vi "DO COUNTER.vi"() -> ()   [LabVIEW 2015]
uses:
  <vilib>/myRIO/Instrument Drivers/Onboard IO/DIO/typedefs/DIO Reference.ctl
  <vilib>/myRIO/Common/Instrument Driver Framework/Utilities/typedefs/myRIO Generic Hardware Reference.ctl
  <vilib>/myRIO/Common/Instrument Driver Framework/Utilities/typedefs/Hardware Version Enum.ctl
  <vilib>/myRIO/Common/Instrument Driver Framework/Utilities/typedefs/myRIO v1.0 Reference.ctl
  <vilib>/myRIO/Common/Instrument Driver Framework/Utilities/typedefs/Generic FPGA Reference.ctl
  <vilib>/myRIO/Common/Instrument Driver Framework/myRIO v1.0/DIO/typedefs/DIO Channels List.ctl
  <vilib>/myRIO/Common/Instrument Driver Framework/myRIO v1.0/DIO/typedefs/DIO Channels Enum.ctl
  <vilib>/userdefined/High Color/nirio_resource_hc.ctl
  <vilib>/myRIO/Common/Instrument Driver Framework/Utilities/vis/Is FPGA Ref Available.vi
  <vilib>/myRIO/Common/Instrument Driver Framework/myRIO v1.0/DIO/vis/myRIO v1.1 Open DIO.vi
  <vilib>/myRIO/Instrument Drivers/Onboard IO/DIO/vis/Write.vi
  <vilib>/myRIO/Common/Instrument Driver Framework/Utilities/vis/Validate Channels.vi
  <vilib>/myRIO/Common/Instrument Driver Framework/myRIO v1.0/DIO/vis/myRIO v1.0 Reserve DIO.vi
  <vilib>/myRIO/Common/Instrument Driver Framework/myRIO v1.0/Resource Manager/vis/myRIO v1.0 Reserve Channel List.vi
  <vilib>/myRIO/Common/Instrument Driver Framework/myRIO v1.0/DIO/vis/myRIO v1.0 Build MUX Configuration DIO.vi
  <vilib>/myRIO/Common/Instrument Driver Framework/myRIO v1.0/Resource Manager/vis/myRIO v1.0 Reserve Channel.vi
  <vilib>/myRIO/Common/Instrument Driver Framework/myRIO v1.0/Resource Manager/vis/myRIO v1.0 Unreserve Channel.vi
  <vilib>/myRIO/Common/Instrument Driver Framework/myRIO v1.0/Resource Manager/vis/myRIO v1.0 Create Configuration List.vi
  <vilib>/myRIO/Common/Instrument Driver Framework/myRIO v1.0/Resource Manager/vis/myRIO v1.0 Build Mutex Name.vi
  <vilib>/Utility/VariantDataType/GetNumericInfo.vi
  <vilib>/Utility/error.llb/Error Cluster From Error Code.vi
  <vilib>/myRIO/Common/Instrument Driver Framework/myRIO v1.0/myRIO v1.1 Open.vi
  <vilib>/myRIO/Common/Instrument Driver Framework/Utilities/vis/IO Manager.vi
  <vilib>/myRIO/Common/Instrument Driver Framework/Utilities/vis/Configuration Manager.vi
  <vilib>/myRIO/Common/Instrument Driver Framework/myRIO v1.0/Resource Manager/vis/myRIO v1.0 Configure IO.vi
  <vilib>/myRIO/Common/Instrument Driver Framework/myRIO v1.0/myRIO v1.0 Close.vi
  <vilib>/myRIO/Common/Instrument Driver Framework/myRIO v1.0/DIO/vis/myRIO v1.0 Write DIO.vi
  <vilib>/myRIO/Express VI/Onboard Devices/LED/LED Express VI.xnode
  <vilib>/myRIO/Instrument Drivers/Onboard IO/DIO/vis/myRIO DIO Open.xnode
  <vilib>/myRIO/Instrument Drivers/Onboard IO/DIO/DIO.lvlib
panel:
  out "C-BINARY":i16[](array[numeric])
  out "C-HEXA":string
  out "C-DEC":u32
  in  "SELECTOR":bool
  out "LED3":bool
  out "LED2":bool
  out "LED1":bool
  in  "Speed":u32 caption="SPEED"
  out "LED0":bool
  # "MSB"
  # "LSB"
  # "MSB"
  # "LSB"
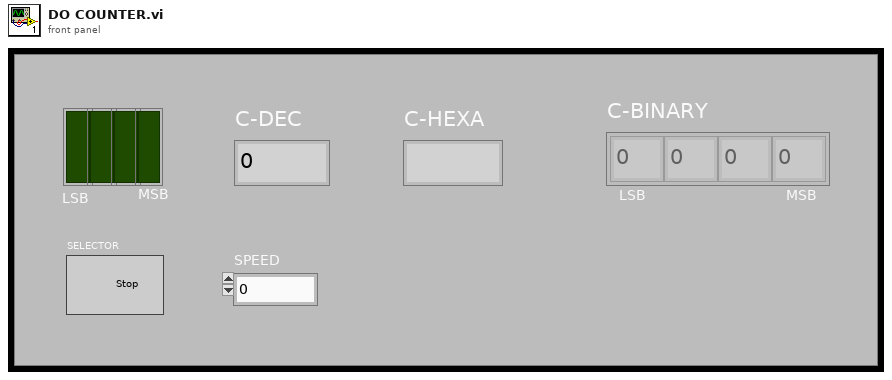
[diagram p1: front panel]
types:
  T1 = typedef "DIO.lvlib/DIO Reference.ctl" = cluster{"myRIO Reference":T2, "DIO Channels List":T6}
  T2 = typedef "myRIO Generic Hardware Reference.ctl" = cluster{"myRIO Model":T3, "myRIO Hardware Reference":T4}
  T3 = typedef "Hardware Version Enum.ctl" = enum16{"Unknown", "myRIO-1900", "myRIO-1950", "roboRIO"}
  T4 = typedef "myRIO v1.0 Reference.ctl" = cluster{"Generic FPGA Reference":T5, "Allow multiple opens":bool}
  T5 = typedef "Generic FPGA Reference.ctl" = refnum<k20>
  T6 = typedef "DIO Channels List.ctl" = T7[]
  T7 = typedef "DIO Channels Enum.ctl" = enum16{"Not Connected", "C/DIO0", "C/DIO1", "C/DIO2", "C/DIO3", "C/DIO4", "C/DIO5", "C/DIO6", "C/DIO7", "A/DIO0", "A/DIO1", "A/DIO2", "A/DIO3", "A/DIO4", "A/DIO5", "A/DIO6", "A/DIO7", "A/DIO8", "A/DIO9", "A/DIO10", "A/DIO11", "A/DIO12", "A/DIO13", "A/DIO14", "A/DIO15", "B/DIO0", "B/DIO1", "B/DIO2", "B/DIO3", "B/DIO4", "B/DIO5", "B/DIO6", "B/DIO7", "B/DIO8", "B/DIO9", "B/DIO10", "B/DIO11", "B/DIO12", "B/DIO13", "B/DIO14", "B/DIO15", "LED0", "LED1", "LED2", "LED3", "Button0", "DIO/DIO0", "DIO/DIO1", "DIO/DIO2", "DIO/DIO3", "DIO/DIO4", "DIO/DIO5", "DIO/DIO6", "DIO/DIO7", "DIO/DIO8", "DIO/DIO9", "SPI/CS0", "SPI/CS1", "SPI/CS2", "SPI/CS3", "LED RADIO (Green)", "LED RADIO (Red)", "LED COMM (Green)", "LED COMM (Red)", "LED MODE (Green)", "LED MODE (Red)"}
  T8 = typedef "nirio_resource_hc.ctl" = tag
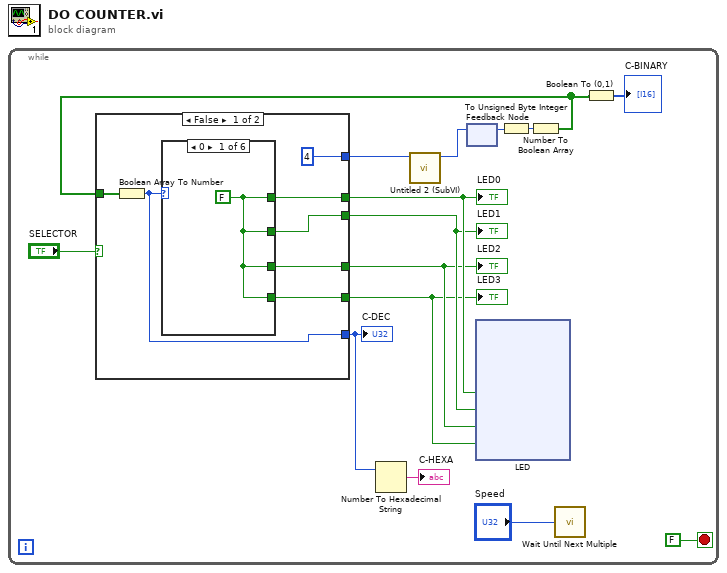
[diagram p0: block diagram]
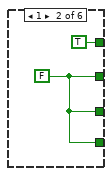
[diagram p2: hidden frame]
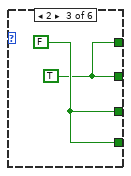
[diagram p3: hidden frame]
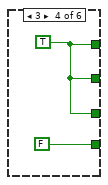
[diagram p4: hidden frame]
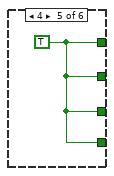
[diagram p5: hidden frame]
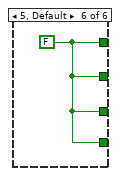
[diagram p6: hidden frame]
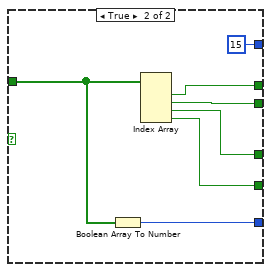
[diagram p7: hidden frame]
diagram:
  n1 = while {
    stop <- FALSE stop-if-true
    n2 = feedback #1() -> (w3:i32)  [unwired: 1 in]
    n3 = To Unsigned Byte Integer(number=w3) -> (unsigned 8bit integer=w13:u8)
    n4 = Number To Boolean Array(number=w13) -> (Boolean array=w1:bool[])
    n5 = case shown="False" "SELECTOR" {
      tunnel: w1 -> [w22 w32]
      tunnel: [w21 w38] -> w12
      tunnel: [w19 w37] -> w11
      tunnel: [w18 w36] -> w10
      tunnel: [w20 w35] -> w9
      tunnel: [4 ("y") 15 ("y")] -> w4
      tunnel: [w16 w33] -> w7
      frame False {
        n6 = Boolean Array To Number(Boolean array=w22) -> (number=w16:u32)
        n7 = case shown="0" w16 {
          tunnel: [w23 TRUE w26 w28 w30 w31] -> w21
          tunnel: [w23 w24 w27 FALSE w30 w31] -> w20
          tunnel: [w23 w24 w26 w28 w30 w31] -> w19
          tunnel: [w23 w24 w27 w28 w30 w31] -> w18
          frame 0 {
            w23 = FALSE
          }
          frame 1 {
            w24 = FALSE
          }
          frame 2 {
            w27 = FALSE
            w26 = TRUE
          }
          frame 3 {
            w28 = TRUE
          }
          frame 4 {
            w30 = TRUE
          }
          frame 5, Default {
            w31 = FALSE
          }
        }
      }
      frame True {
        n8 = Boolean Array To Number(Boolean array=w32) -> (number=w33:u32)
        n9 = Index Array(array=w32) -> (element #1=w38:bool, element #2=w37:bool, element #3=w36:bool, element #4=w35:bool)  [unwired: 4 in]
      }
    }
    "LED0" <- w12
    "LED2" <- w10
    "LED3" <- w9
    "LED1" <- w11
    "C-DEC" <- w7
    n10 = Number To Hexadecimal String(2:w7) -> (0:→"C-HEXA":string)  [unwired: 1 in]
    n11 = call "Untitled 2 (SubVI).vi"("y"=w4) -> ("Numeric"=w2:i32)  [unwired: 9 in, 1 out]
    n12 = feedback-in #1(w2) -> ()
    n13 = xnode "LED"("LED0"=w12, "LED1"=w11, "LED2"=w10, "LED3"=w9) -> ()  [unwired: 1 in, 1 out]
    n14 = call "Wait Until Next Multiple"("Count(mSec)"="Speed") -> ()  [unwired: 1 out]
    n15 = Boolean To (0,1)(Boolean=w1) -> (0, 1=→"C-BINARY":i16[])
  }
